vi "Open VISA Port for Arduino.vi"(8 "error in (no error)":errorcluster, 10 "baud rate (9600)":u32=9600, 11 "VISA resource name":refnum<visa-resource-name>) -> (0 "error out":errorcluster, 3 "VISA resource name out":refnum<visa-resource-name>)   [LabVIEW 2024, in "FW Arduino Control.lvclass"]
uses:
  FW Arduino Control.lvclass
  531df36b-102b-49fc-b73d-50a8115d9375.vi
  <vilib>/Instr/_visa.llb/VISA Configure Serial Port (Instr).vi
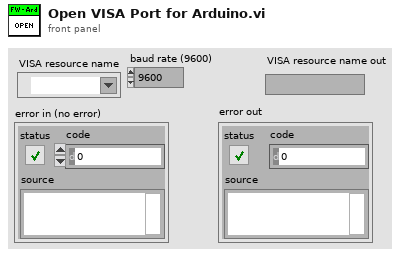
[diagram p1: front panel]
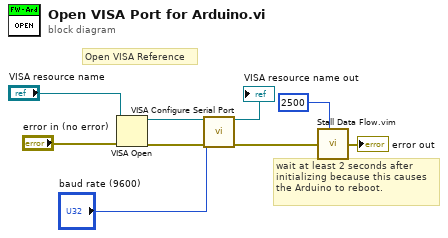
[diagram p0: block diagram]
diagram:
  # "wait at least 2 seconds after initializing because this causes the Arduino to reboot."
  # "Open VISA Reference"
  n1 = VISA Open(error in (no error)="error in (no error)", VISA resource name="VISA resource name") -> (VISA resource name=w6:refnum<visa-resource-name>, error out=w7:errorcluster)  [unwired: 3 in]
  n2 = call-poly "VISA Configure Serial Port"("VISA resource name"=w6, "baud rate (9600)"="baud rate (9600)", "error in (no error)"=w7) -> ("VISA resource name out"=→"VISA resource name out":refnum<visa-resource-name>, "error out"=w8:errorcluster)  [unwired: 11 in]
  n3 = call "Stall Data Flow.vim"("value in"=w8, "milliseconds to wait"=u32 2500) -> ("value out"=→"error out":errorcluster)  [unwired: 1 out]
